vi "Gyro test.vi"() -> ()   [LabVIEW 2012, in "Compass IO.lvlib"]
uses:
  Compass IO.lvlib
  <vilib>/Platform/TimedLoop/XDataNode/timing_clust.ctl
  <vilib>/Platform/TimedLoop/XDataNode/nitl_modes.ctl
  <vilib>/Platform/TimedLoop/XDataNode/wakeup.ctl
  <vilib>/FPGAPlugInAG/sbRIO-9636/niLvFpga_Open_sbRIO-9636.vi
  <vilib>/rvi/interface/common/dynamic/niFpgaDynamicAddResources.vi
  <vilib>/FPGAPlugInAG/Dynamic/niLvFpga_Close_Dynamic.vi
  <vilib>/platform/TimedLoop/XDataNode/XDataNode.xnode
  <vilib>/rvi/interface/nirviOpenFPGA/nirviOpenFPGA.xnode
  FPGA Bitfiles/NIARC_FPGATarget_FPGACompile_e4XhunWUay0.lvbitx
  <vilib>/rvi/interface/nirviCloseFPGA/nirviCloseFPGA.xnode
  <vilib>/IEDriver/SPIandI2C/Host/I2C/I2C Host.lvlib
  <vilib>/Platform/TimedLoop/XDataNode/XDNodeRunTimeDep.lvlib
panel:
  out "Waveform Graph":dbl[](graph)
  out "z":i16
  out "y":i16
  out "x":i16
  in  "stop":bool
  out "Data":u8[](array[numeric])
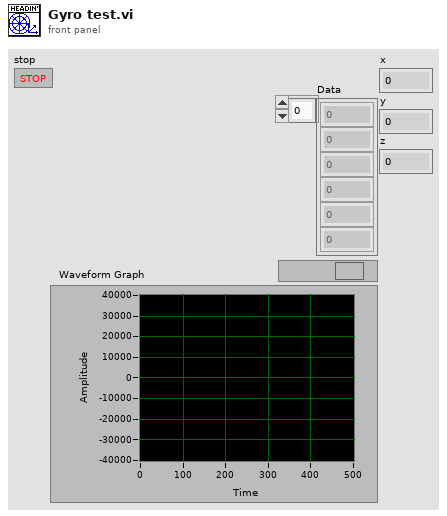
[diagram p1: front panel]
types:
  T1 = cluster{"FPGA VI Reference":refnum<k20>, "Port Number":u8}
  T2 = typedef "XDNodeRunTimeDep.lvlib/timing_clust.ctl" = cluster{"Expected End [f-1]":u64, "Actual End [f-1]":u64, "Finished Late? [f-1]":bool, "Expected End [i-1]":u64, "Actual End [i-1]":u64, "Finished Late? [i-1]":bool, "Expected Start [i]":u64, "Actual Start [i]":u64, "Expected Start [f]":u64, "Actual Start [f]":u64, "Source Name":string, "Structure Name":string, "Period":i64, "Deadline":i64, "Offset":i64, "Start":i64, "Priority":i32, "Timeout":i32, "Mode":T3, "Wakeup Reason":T4, "Error":errorcluster, "Source Type":string, "Secondary Source Type":string, "Global End Time":u64, "Global Start Time":u64, "Frame Duration":u64, "Iteration Duration":u64, "Assigned CPU":i32, "I/O Scan Engine Mode":u32}
  T3 = typedef "XDNodeRunTimeDep.lvlib/nitl_modes.ctl" = enum32{"No Change", "Process missed periods, maintain original phase", "Discard missed periods, maintain original phase", "Process missed periods, ignore original phase", "Discard missed periods, ignore original phase"}
  T4 = typedef "XDNodeRunTimeDep.lvlib/wakeup.ctl" = enum32{"Normal", "Aborted", "Asynchronous wakeup", "Timing source error", "Timed loop error", "Timeout"}
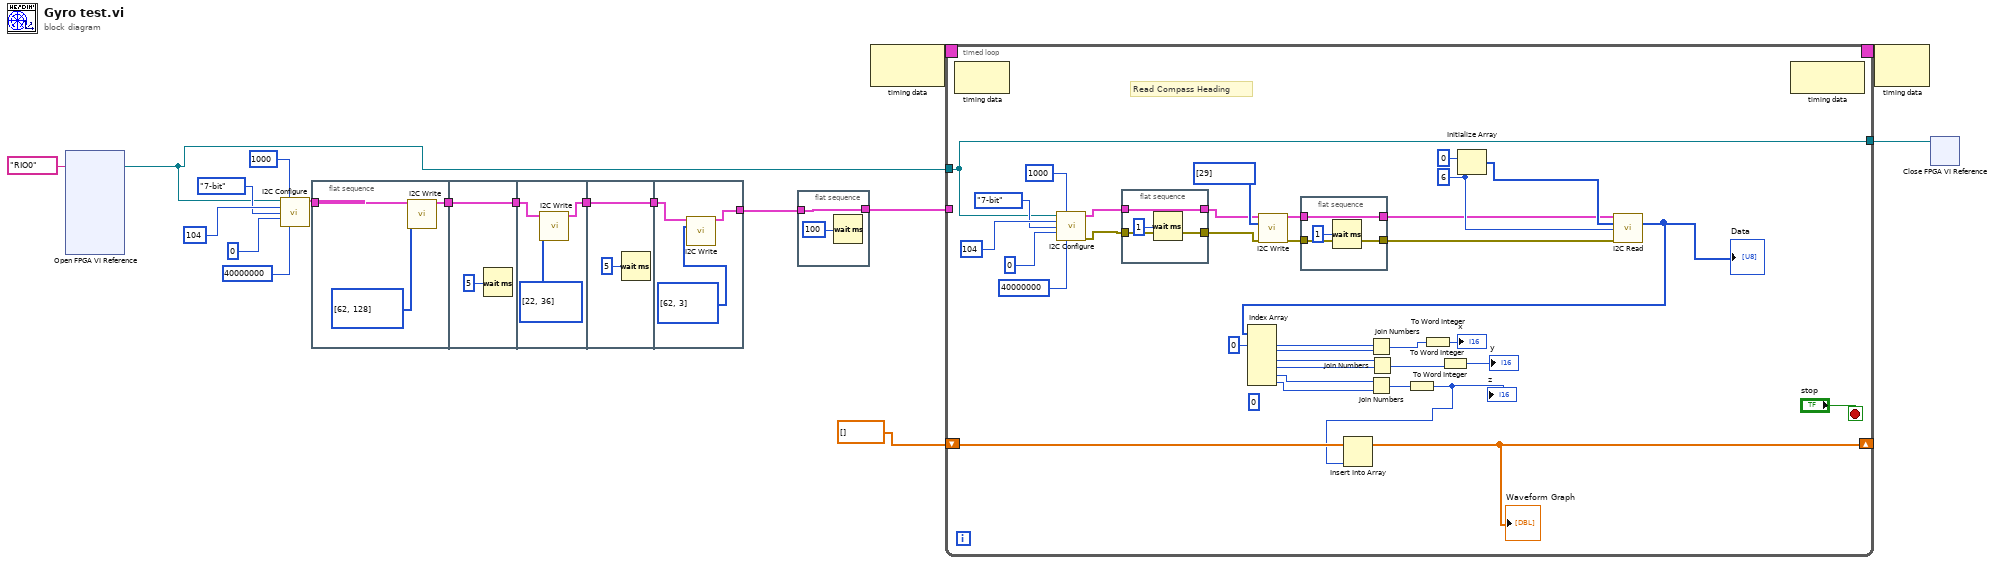
[diagram p0: block diagram]
diagram:
  n1 = xnode "Open FPGA VI Reference"("resource name"=tag "RIO0") -> ("FPGA VI Reference Out"=w10:refnum<k20>)  [unwired: 1 in, 1 out]
  n2 = call <vilib>:"I2C Configure.vi"("FPGA VI Reference"=w10, "Clock Rate"=u32 1000, "Address"=u16 104, "Address Type (7-bit)"=enum16{"7-bit", "10-bit"}."7-bit", "Port Number"=u8 0, "FPGA Clock (40 MHz)"=u32 40000000 ("Clock Rate")) -> ("FPGA Information Out"=w9:T1)  [unwired: 8 in, 1 out]
  n3 = flat-sequence {
    tunnel: w9 -> [w21]
    tunnel: [w19] -> w7
    tunnel: w7 -> [w23]
    tunnel: [w23] -> w6
    tunnel: w6 -> [w25]
    tunnel: [w24] -> w5
    tunnel: w5 -> [w28]
    tunnel: [w28] -> w4
    tunnel: w4 -> [w30]
    tunnel: [w29] -> w2
    frame #0 {
      n4 = call <vilib>:"I2C Write.vi"("FPGA Information In"=w21, "Data"=u8[] [62, 128]) -> ("FPGA Information Out"=w19:T1)  [unwired: 12 in, 1 out]
    }
    frame #1 {
      n5 = Wait (ms)(milliseconds to wait=u32 5) -> ()  [unwired: 1 out]
    }
    frame #2 {
      n6 = call <vilib>:"I2C Write.vi"("FPGA Information In"=w25, "Data"=u8[] [22, 36]) -> ("FPGA Information Out"=w24:T1)  [unwired: 12 in, 1 out]
    }
    frame #3 {
      n7 = Wait (ms)(milliseconds to wait=u32 5) -> ()  [unwired: 1 out]
    }
    frame #4 {
      n8 = call <vilib>:"I2C Write.vi"("FPGA Information In"=w30, "Data"=u8[] [62, 3]) -> ("FPGA Information Out"=w29:T1)  [unwired: 12 in, 1 out]
    }
  }
  n9 = flat-sequence {
    tunnel: [w32] -> w3
    tunnel: w2 -> [w32]
    frame #0 {
      n10 = Wait (ms)(milliseconds to wait=u32 100) -> ()  [unwired: 1 out]
    }
  }
  n11 = node-c288() -> (w17:T2)  [unwired: 1 in]
  n12 = timed-loop {
    timing: w17 -> [_]
    timing-out: [_] -> w16
    tunnel: w10 -> [w54]
    tunnel: [w54] -> w8
    tunnel: w3 -> [_]
    shift-right: [w38] -> _
    shift-left: dbl[] [] ("array") -> [w40]
    stop <- "stop" stop-if-true
    (unwired) 0
    w59 = u16 6 ("dimension size")
    # "Read Compass Heading"
    n13 = node-c288() -> ()  [unwired: 1 in, 1 out]
    n14 = call <vilib>:"I2C Configure.vi"("FPGA VI Reference"=w54, "Clock Rate"=u32 1000, "Address"=u16 104, "Address Type (7-bit)"=enum16{"7-bit", "10-bit"}."7-bit", "Port Number"=u8 0, "FPGA Clock (40 MHz)"=u32 40000000 ("Clock Rate")) -> ("FPGA Information Out"=w37:T1, "error out"=w36:errorcluster)  [unwired: 8 in]
    n15 = flat-sequence {
      tunnel: w37 -> [w71]
      tunnel: w36 -> [w70]
      tunnel: [w71] -> w35
      tunnel: [w70] -> w34
      frame #0 {
        n16 = Wait (ms)(milliseconds to wait=u32 1) -> ()  [unwired: 1 out]
      }
    }
    n17 = call <vilib>:"I2C Write.vi"("FPGA Information In"=w35, "Data"=u8[] [29], "error in (no error)"=w34) -> ("FPGA Information Out"=w58:T1, "error out"=w57:errorcluster)  [unwired: 11 in]
    n18 = flat-sequence {
      tunnel: w58 -> [w74]
      tunnel: w57 -> [w73]
      tunnel: [w74] -> w56
      tunnel: [w73] -> w55
      frame #0 {
        n19 = Wait (ms)(milliseconds to wait=u32 1) -> ()  [unwired: 1 out]
      }
    }
    n20 = Initialize Array(u8 0 ("element"), w59) -> (w60:u8[])
    n21 = call <vilib>:"I2C Read.vi"("FPGA Information In"=w56, "Input Array"=w60, "Number of Bytes to Read"=w59, "error in (no error)"=w55) -> ("Data"=w53:u8[])  [unwired: 9 in, 2 out]
    "Data" <- w53
    n22 = Index Array(array=w53, index #1=0 ("index")) -> (element #1=w51:u8, element #2=w43:u8, element #3=w50:u8, element #4=w42:u8, element #5=w49:u8, element #6=w41:u8)  [unwired: 5 in]
    n23 = Join Numbers(hi=w51, lo=w43) -> ((hi.lo)=w48:u16)
    n24 = Join Numbers(hi=w49, lo=w41) -> ((hi.lo)=w46:u16)
    n25 = Join Numbers(hi=w50, lo=w42) -> ((hi.lo)=w47:u16)
    n26 = To Word Integer(number=w46) -> (16bit integer=w39:i16)
    "z" <- w39
    n27 = Insert Into Array(array=w40, new element=w39) -> (w38:dbl[])  [unwired: 1 in]
    "Waveform Graph" <- w38
    n28 = To Word Integer(number=w48) -> (16bit integer=→"x":i16)
    n29 = To Word Integer(number=w47) -> (16bit integer=→"y":i16)
    n30 = node-c288() -> ()  [unwired: 1 in, 1 out]
  }
  n31 = node-c288(w16) -> ()  [unwired: 1 out]
  n32 = xnode "Close FPGA VI Reference"("FPGA VI Reference In"=w8) -> ()  [unwired: 1 in, 1 out]
